vi "SimuladorTemp.vi"(10 "Lmin":dbl, 11 "Lmax":dbl) -> (3 "Numeric":dbl)   [LabVIEW 2020]
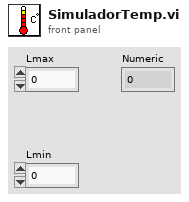
[diagram p1: front panel]
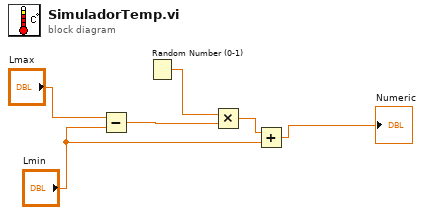
[diagram p0: block diagram]
diagram:
  n1 = Subtract(x="Lmax", y="Lmin") -> (x-y=w3:dbl)
  n2 = Random Number (0-1)() -> (number: 0 to 1=w2:dbl)
  n3 = Multiply(x=w2, y=w3) -> (x*y=w4:dbl)
  n4 = Add(x=w4, y="Lmin") -> (x+y=→"Numeric":dbl)
